vi "Execute_Row.vi"(3 "Simulate/Run":T2, 5 "Traverse line":T3 {"Carrier_2 Q (l/min)" format="%#.2f"; "Row Duration (mins)" format="%#.1f"; "Row No" min=0; "Trace Gas Concentration (%)" min=0.0 format="%#_4f"; "Carrier_1 Q (l/min)" format="%#.2f"; "Tunnel Speed" format="%#.2f"; "Start X" format="%#.2f"; "Start Y" format="%#.2f"; "Start Z" format="%#.2f"; "End X" format="%#.2f"; "End Y" format="%#.2f"; "End Z" format="%#.2f"; "Averaging time (min)" min=0.0 format="%#.2f"}) -> (1 "Status":T1, 2 "Traverse line out":T3 {"Carrier_2 Q (l/min)" format="%#.2f"; "Row Duration (mins)" format="%#.1f"; "Row No" min=0; "Trace Gas Concentration (%)" min=0.0 format="%#_4f"; "Carrier_1 Q (l/min)" format="%#.2f"; "Tunnel Speed" format="%#.2f"; "Start X" format="%#.2f"; "Start Y" format="%#.2f"; "Start Z" format="%#.2f"; "End X" format="%#.2f"; "End Y" format="%#.2f"; "End Z" format="%#.2f"; "Averaging time (min)" min=0.0 format="%#.2f"})   [LabVIEW 2015]
uses:
  Traverse_cluster.ctl
  Spacing.ctl
  Controls/Multi_run_mode.ctl
  Controls/User_Specific_mode.ctl
  Multi_Run_Status.ctl
  Controls/Setup.ctl
  Controls/Save_Data.ctl
  Globals/Constants_global.vi
  Globals/Extra_Commands_Global.vi
  Globals/Trav_pos_global.vi
panel:
  # "X           Y            Z"
  # "Start"
  # "End"
  # "X           Y            Z"
  # "Start"
  # "End"
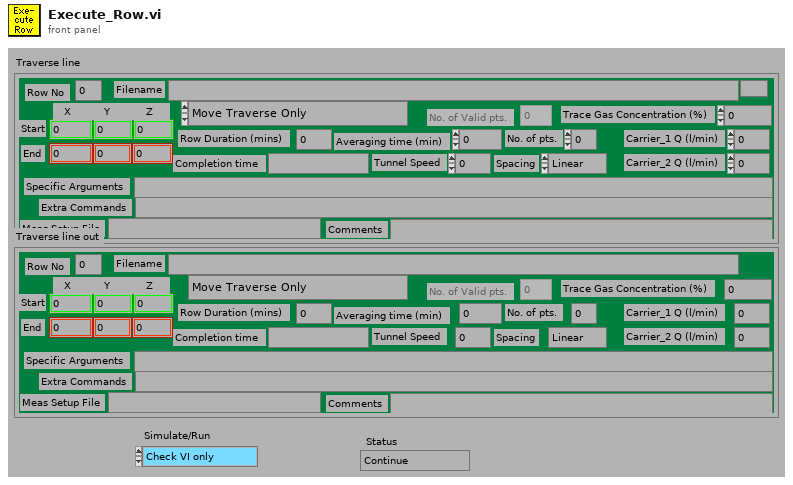
[diagram p1: front panel]
types:
  T1 = typedef "Multi_Run_Status.ctl" = enum16{"Continue", "Jump to Next Point", "Jump to Next Row", "Jump To Fall Back", "Terminate Run"}
  T2 = typedef "User_Specific_mode.ctl" = enum16{"Check VI only", "Run VI"}
  T3 = typedef "Traverse_cluster.ctl" = cluster{"Start X":sgl, "Start Y":sgl, "Start Z":sgl, "End X":sgl, "End Y":sgl, "End Z":sgl, "No. of pts.":i32, "Spacing":T4, "Filename":path, "Tunnel Speed":dbl, "Averaging time (min)":dbl, "Extra Commands":string, "Carrier_1 Q (l/min)":dbl, "Carrier_2 Q (l/min)":dbl, "Trace Gas Concentration (%)":dbl, "Specific Arguments":string, "Comments":string, "Row No":i32, "Row Type Selector":T5, "Completion time":string, "Row Duration (mins)":dbl, "No. of Valid pts.":i32, "Meas Setup File":string}
  T4 = typedef "Spacing.ctl" = enum16{"Linear", "Log", "Gauss", "Specified", "N/A"}
  T5 = typedef "Multi_run_mode.ctl" = enum16{"Move Traverse Only", "Set Tunnel Speed Only", "Set Source Only", "Set Measurement Conditions", "Single Measurement", "Vertical Profile", "Lateral Profile", "Longitudinal Profile", "Explore Volume", "Multi-Axis Profile", "Auto Calibrate", "Meas Fast FID Bkgnd", "Check Beam Power", "Scanning Valve Measurement", "Run VI Named:", "Set ADAM Ch", "Wait (minutes)", "Send Message", "Synchronize With:", "Fall Back to this Row", "Turn Off Row Repeating", "Blank Row", "Traverse 3D Volume"}
  T6 = typedef "Save_Data.ctl" = enum16{"Save No Data", "Save Data"}
  T7 = typedef "Setup.ctl" = enum16{"Run Program", "Show Setup", "Save Current Setup", "Setup Front Panel"}
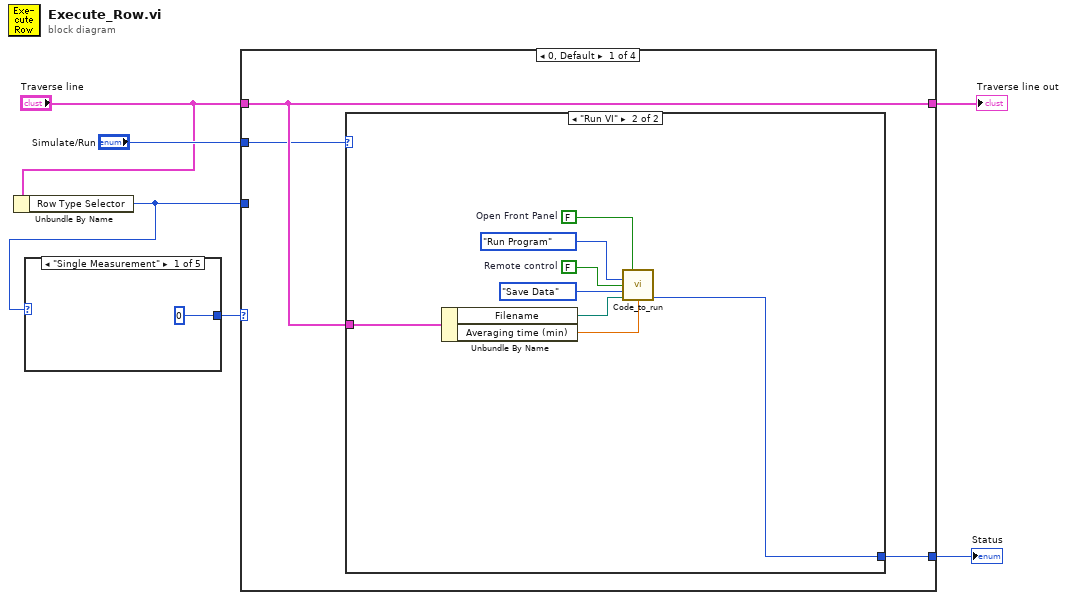
[diagram p0: block diagram]
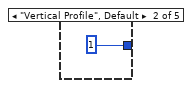
[diagram p2: hidden frame]
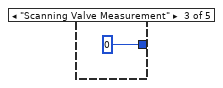
[diagram p3: hidden frame]
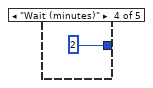
[diagram p4: hidden frame]
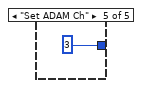
[diagram p5: hidden frame]
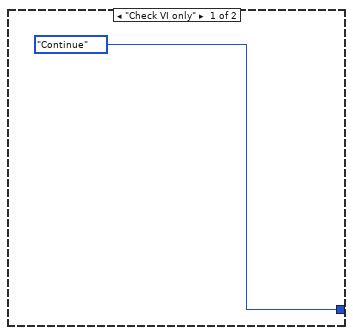
[diagram p6: hidden frame]
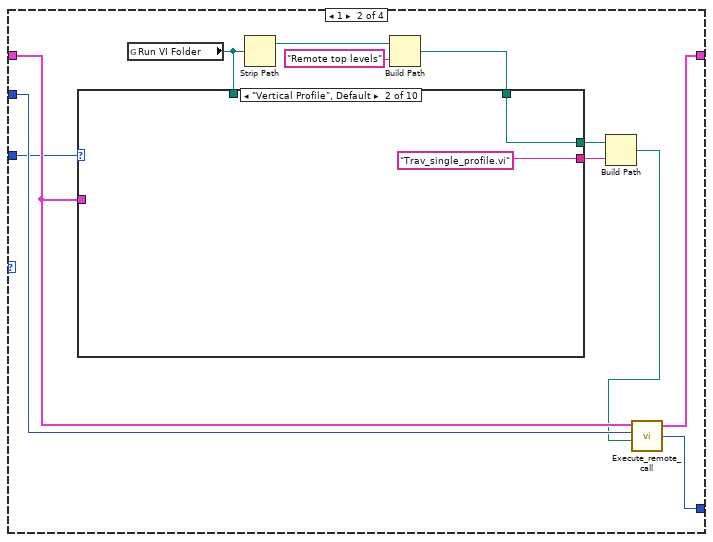
[diagram p7: hidden frame]
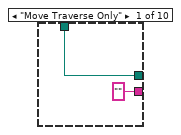
[diagram p8: hidden frame]
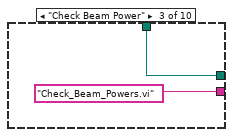
[diagram p9: hidden frame]
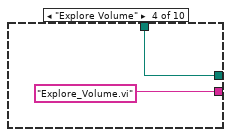
[diagram p10: hidden frame]
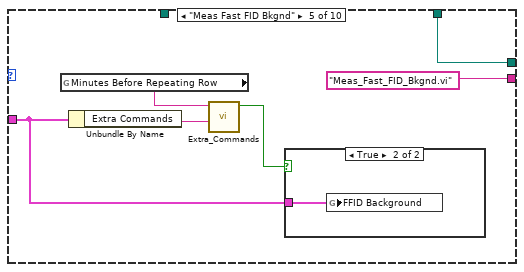
[diagram p11: hidden frame]
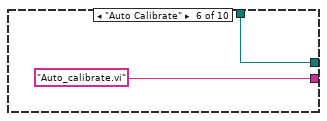
[diagram p13: hidden frame]
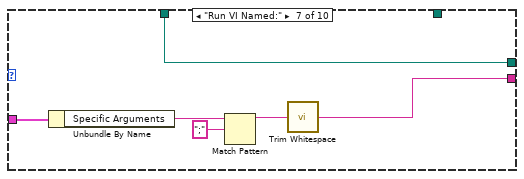
[diagram p14: hidden frame]
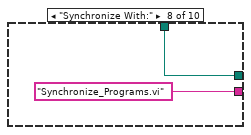
[diagram p15: hidden frame]
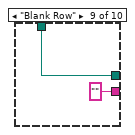
[diagram p16: hidden frame]
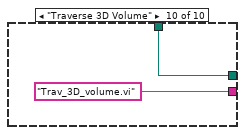
[diagram p17: hidden frame]
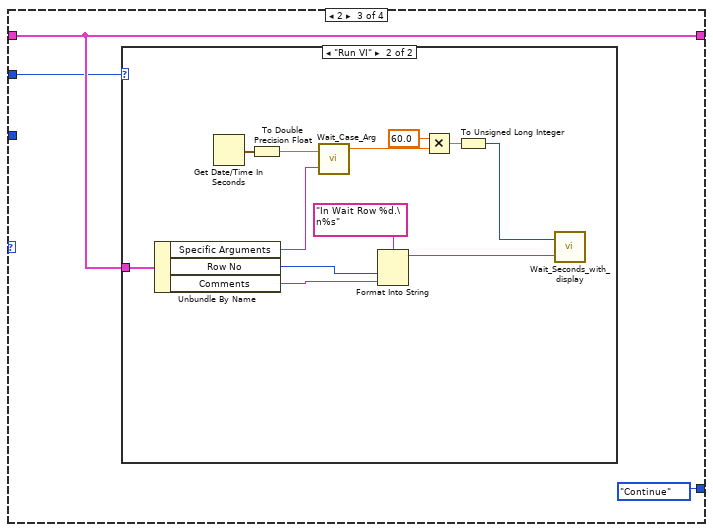
[diagram p18: hidden frame]
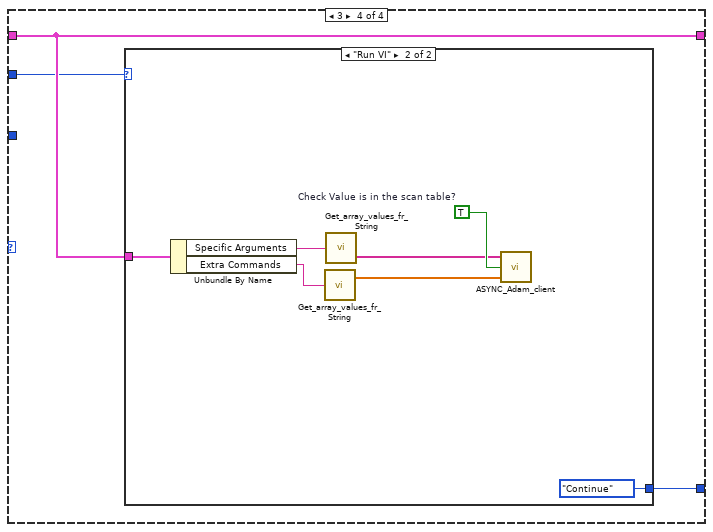
[diagram p20: hidden frame]
diagram:
  n1 = Unbundle By Name("Traverse line") -> ("Row Type Selector"=w2:T5)
  n2 = case shown="\"Single Measurement\"" w2 {
    tunnel: [0 1 0 2 3] -> w3
    frame "Single Measurement" {
    }
    frame "Vertical Profile", Default {
    }
    frame "Scanning Valve Measurement" {
    }
    frame "Wait (minutes)" {
    }
    frame "Set ADAM Ch" {
    }
  }
  n3 = case shown="0, Default" w3 {
    tunnel: [w14 w31 Multi_Run_Status."Continue" ("Status") w82] -> w1
    tunnel: "Traverse line" -> [w13 w33 w67 w81]
    tunnel: [w13 w35 w67 w81] -> w6
    tunnel: "Simulate/Run" -> [w12 w34 w65 w80]
    tunnel: w2 -> [_ w32 _ _]
    frame 0, Default {
      n4 = case shown="\"Run VI\"" w12 {
        tunnel: [Multi_Run_Status."Continue" ("Status") w23] -> w14
        tunnel: w13 -> [_ w22]
        frame "Check VI only" {
        }
        frame "Run VI" {
          w18 = FALSE  # Open Front Panel
          w20 = FALSE  # Remote control
          n5 = Unbundle By Name(w22) -> ("Filename"=w21:path, "Averaging time (min)"=w19:dbl)
          n6 = call "Code_to_run.vi"("Open Front Panel"=w18, "setup"=Setup."Run Program", "Remote control"=w20, "File"=Save_Data."Save Data", "Results Filename"=w21, "Averaging time (min)"=w19) -> ("Status"=w23:T1)  [unwired: 5 in, 4 out]
        }
      }
    }
    frame 1 {
      n7 = global read "Constants_global.vi" "Run VI Folder"() -> (w24:path)
      n8 = Strip Path(path=w24) -> (stripped path=w25:path)  [unwired: 1 out]
      n9 = Build Path(base path=w25, name or relative path="Remote top levels") -> (appended path=w29:path)
      n10 = case shown="\"Vertical Profile\", Default" w32 {
        tunnel: w29 -> [w37 w39 w41 w43 w49 w52 _ w60 w62 w64]
        tunnel: w33 -> [_ _ _ _ w44 _ w58 _ _ _]
        tunnel: [w37 w39 w41 w43 w49 w52 w57 w60 w62 w64] -> w28
        tunnel: ["" ("name") "Trav_single_profile.vi" "Check_Beam_Powers.vi" "Explore_Volume.vi" "Meas_Fast_FID_Bkgnd.vi" "Auto_calibrate.vi" w53 "Synchronize_Programs.vi" "" ("name") "Trav_3D_volume.vi" ("name")] -> w27
        tunnel: w24 -> [_ _ _ _ _ _ w57 _ _ _]
        frame "Move Traverse Only" {
        }
        frame "Vertical Profile", Default {
        }
        frame "Check Beam Power" {
        }
        frame "Explore Volume" {
        }
        frame "Meas Fast FID Bkgnd" {
          n11 = global read "Extra_Commands_Global.vi" "Minutes Before Repeating Row"() -> (w47:string)
          n12 = Unbundle By Name(w44) -> ("Extra Commands"=w46:string)
          n13 = call "Extra_Commands.vi"("String to Search"=w46, "Command"=w47) -> ("Command Found"=w45:bool)  [unwired: 1 in, 4 out]
          n14 = case shown="True" w45 {
            tunnel: w44 -> [_ w50]
            frame False {
            }
            frame True {
              n15 = global write "Trav_pos_global.vi" "FFID Background"(w50) -> ()
            }
          }
        }
        frame "Auto Calibrate" {
        }
        frame "Run VI Named:" {
          n16 = Unbundle By Name(w58) -> ("Specific Arguments"=w55:string)
          n17 = Match Pattern(string=w55, regular expression=";") -> (before substring=w54:string)  [unwired: 4 out]
          n18 = call <vilib>:"Trim Whitespace.vi"("string"=w54) -> ("trimmed string"=w53:string)  [unwired: 1 in]
        }
        frame "Synchronize With:" {
        }
        frame "Blank Row" {
        }
        frame "Traverse 3D Volume" {
        }
      }
      n19 = Build Path(base path=w28, name or relative path=w27) -> (appended path=w26:path)
      n20 = call "Execute_remote_call.vi"("Traverse line"=w33, "Simulate/Run"=w34, "VI to run"=w26) -> ("Traverse Out"=w35:T3, "Status"=w31:T1)  [unwired: 1 in, 3 out]
    }
    frame 2 {
      n21 = case shown="\"Run VI\"" w65 {
        tunnel: w67 -> [_ w73]
        frame "Check VI only", Default {
        }
        frame "Run VI" {
          n22 = Unbundle By Name(w73) -> ("Specific Arguments"=w74:string, "Row No"=w69:i32, "Comments"=w68:string)
          n23 = Get Date/Time In Seconds() -> (seconds since 1Jan1904=w72:timestamp)
          n24 = To Double Precision Float(number=w72) -> (double precision float=w75:dbl)
          n25 = call "Wait_Case_Arg.vi"("Specific Argument"=w74, "seconds since 1Jan1904"=w75) -> ("Minutes To Wait"=w76:dbl)  [unwired: 4 out]
          n26 = Format Into String(format string="In Wait Row %d.\n%s", w69, w68) -> (resulting string=w71:string)  [unwired: 2 in, 1 out]
          n27 = Multiply(x=60.0, y=w76) -> (x*y=w77:dbl)
          n28 = To Unsigned Long Integer(number=w77) -> (unsigned 32bit integer=w78:u32)
          n29 = call "Wait_Seconds_with_display.vi"("Message"=w71, "Seconds to wait"=w78) -> ()  [unwired: 2 out]
        }
      }
    }
    frame 3 {
      n30 = case shown="\"Run VI\"" w80 {
        tunnel: [Multi_Run_Status."Continue" ("Status") Multi_Run_Status."Continue" ("Status")] -> w82
        tunnel: w81 -> [_ w90]
        frame "Check VI only" {
        }
        frame "Run VI" {
          w88 = TRUE  # Check Value is in the scan table?
          n31 = Unbundle By Name(w90) -> ("Specific Arguments"=w87:string, "Extra Commands"=w85:string)
          n32 = call "Get_array_values_fr_String.vi"("String Value"=w85) -> ("Numeric Array"=w84:dbl[])  [unwired: 1 out]
          n33 = call "Get_array_values_fr_String.vi"("String Value"=w87) -> ("String array"=w86:string[])  [unwired: 1 out]
          n34 = call "ASYNC_Adam_client.vi"("Values"=w84, "Check Value is in the scan table?"=w88, "Channel Names"=w86) -> ()  [unwired: 2 out]
        }
      }
    }
  }
  "Traverse line out" <- w6
  "Status" <- w1
